vi "Chunk1DArray.vi"(1 "Chunk Size":i32=2, 2 "1D Array":i32[](array[numeric])) -> (0 "Chunked 2D Array":i32[][](array[numeric]))   [LabVIEW 2014, in "navX-MXP IMU.lvlib"]
uses:
  navX-MXP IMU.lvlib
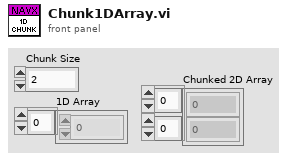
[diagram p1: front panel]
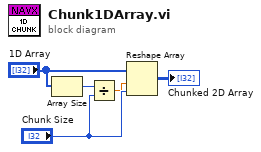
[diagram p0: block diagram]
diagram:
  n1 = Array Size(array="1D Array") -> (size(s)=w5:i32)
  n2 = Divide(x=w5, y="Chunk Size") -> (x/y=w3:dbl)
  n3 = Reshape Array("1D Array", w3, "Chunk Size") -> (→"Chunked 2D Array":i32[][])
